vi "SVFA Convert Frequency (CPM to CPS).vi"(5 "nominal speed [RPM]":dbl=100.0) -> (1 "frequency [Hz]":dbl)   [LabVIEW 2017]
doc: "Converts the unit of a rotational speed from revolutions per minute to revolutions per second, or hertz."
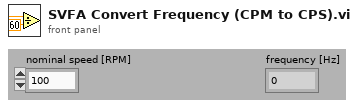
[diagram p1: front panel]
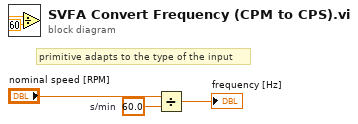
[diagram p0: block diagram]
diagram:
  w2 = 60.0  # s/min
  # "primitive adapts to the type of the input"
  n1 = Divide(x="nominal speed [RPM]", y=w2) -> (x/y=→"frequency [Hz]":dbl)
